vi "Write element.vi"(8 "error in":errorcluster, 10 "element":i32, 11 "EIP Tags Channel in":refnum<class "EIP Tags Channel.lvclass">) -> (0 "error out":errorcluster, 3 "EIP Tags Channel out":refnum<class "EIP Tags Channel.lvclass">)   [LabVIEW 2013, in "EIP Tags Channel.lvclass"]
uses:
  EIP Tags Channel.lvclass
  EIP Tags Channel.lvclass/EIP Tags Channel.ctl
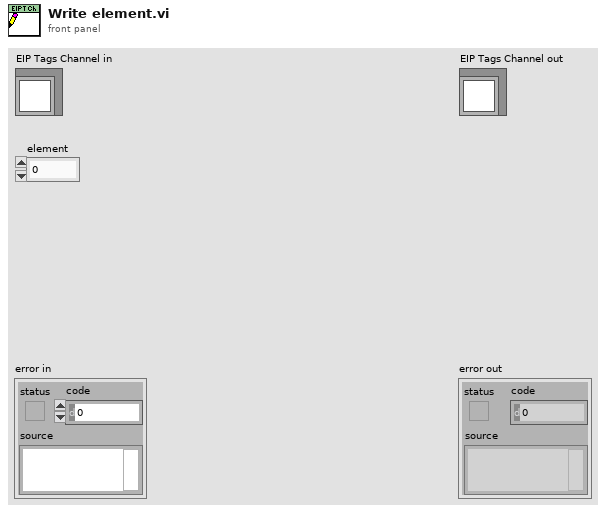
[diagram p1: front panel]
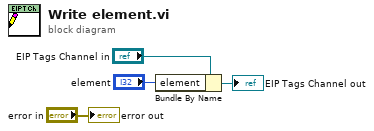
[diagram p0: block diagram]
diagram:
  n1 = Bundle By Name(cluster="EIP Tags Channel in", "element"="element") -> (→"EIP Tags Channel out":refnum<class "EIP Tags Channel.lvclass">)
  "error out" <- "error in"
